vi "setGrid.vi"(0 "reference":refnum<class "Grid.lvclass">, 1 "gridX":dbl format="%.2f", 2 "gridY":dbl format="%.2f", 5 "error in (no error)":errorcluster) -> (14 "reference out":refnum<class "Grid.lvclass">, 19 "error out":errorcluster)   [LabVIEW 2016, in "Grid.lvclass"]
doc: "public void setGrid(double x, double y)"
uses:
  <resource>/Framework/Providers/Open_GDS/UML/Grid_class/Grid.lvclass
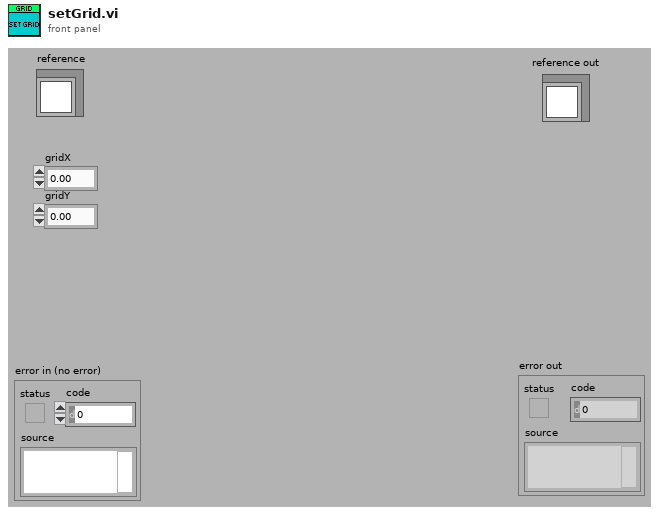
[diagram p1: front panel]
types:
  T1 = typedef "Grid.lvclass/ObjectAttributes.ctl" = cluster{"gridX":dbl, "gridY":dbl, "gridColor":u32}
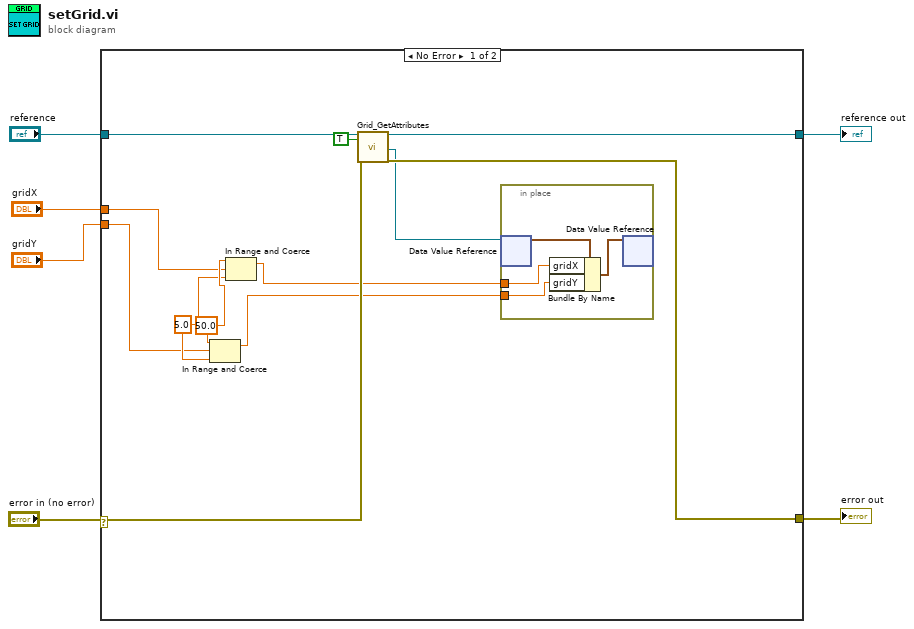
[diagram p0: block diagram]
diagram:
  n1 = case shown="No Error" "error in (no error)" {
    selector: "error in (no error)" -> [w15 w23]
    tunnel: "reference" -> [w18 w24]
    tunnel: [w17 w23] -> w5
    tunnel: [w16 w24] -> w4
    tunnel: "gridX" -> [w12 _]
    tunnel: "gridY" -> [w11 _]
    frame No Error {
      w14 = 50.0 ("upper limit")
      w13 = 5.0 ("lower limit")
      n2 = In Range and Coerce(upper limit=w14, x=w11, lower limit=w13) -> (coerced(x)=w7:dbl)  [unwired: 1 out]
      n3 = In Range and Coerce(upper limit=w14, x=w12, lower limit=w13) -> (coerced(x)=w8:dbl)  [unwired: 1 out]
      n4 = call <resource>:"Grid_GetAttributes.vi"("reference in"=w18, "OnlyGetDvrReference(False)"=TRUE, "error in (no error)"=w15) -> ("reference out"=w16:refnum<class "Grid.lvclass">, "DataRef"=w9:refnum<data-value>, "error out"=w17:errorcluster)  [unwired: 13 in, 1 out]
      n5 = in-place {
        in-place-border: w8 -> [w21]
        in-place-border: w7 -> [w20]
        n6 = in-place-dvr #1(w9) -> (w22:T1)  [unwired: 1 out]
        n7 = Bundle By Name(cluster=w22, "gridX"=w21, "gridY"=w20) -> (w19:T1)
        n8 = in-place-dvr #1(w19) -> ()  [unwired: 2 out]
      }
    }
    frame Error {
    }
  }
  "reference out" <- w4
  "error out" <- w5
